vi "ADAM_Comparitor.vi"(3 "Comparator Info":T1, 4 "Ch names":string[](array[string]), 5 "Present scan array":dbl[](array[numeric]) format="%.2f") -> (0 "Comparator Info Out":T1, 2 "Scan comment":string)   [LabVIEW 2010]
uses:
  ADAM_Comparitor.ctl
  ADAM Client/Sub VIs/ADAM Controls/Search_mode.ctl
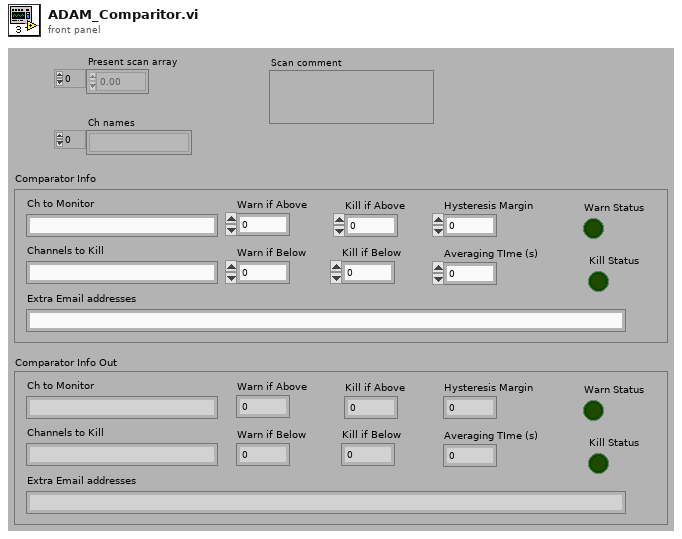
[diagram p1: front panel]
types:
  T1 = typedef "ADAM_Comparitor.ctl" = cluster{"Ch to Monitor":string, "Channels to Kill":string, "Warn if Above":dbl, "Warn if Below":dbl, "Kill if Above":dbl, "Kill if Below":dbl, "Hysteresis Margin":dbl, "Averaging TIme (s)":dbl, "Warn Status":bool, "Kill Status":bool, "Extra Email addresses":string}
  T2 = typedef "Search_mode.ctl" = enum16{"Between times", "All Times"}
  T3 = cluster{"Centre Times":dbl[], "Output array":dbl[]}
  T4 = cluster{"Centre Times":dbl[], "Output array":dbl[]}[]
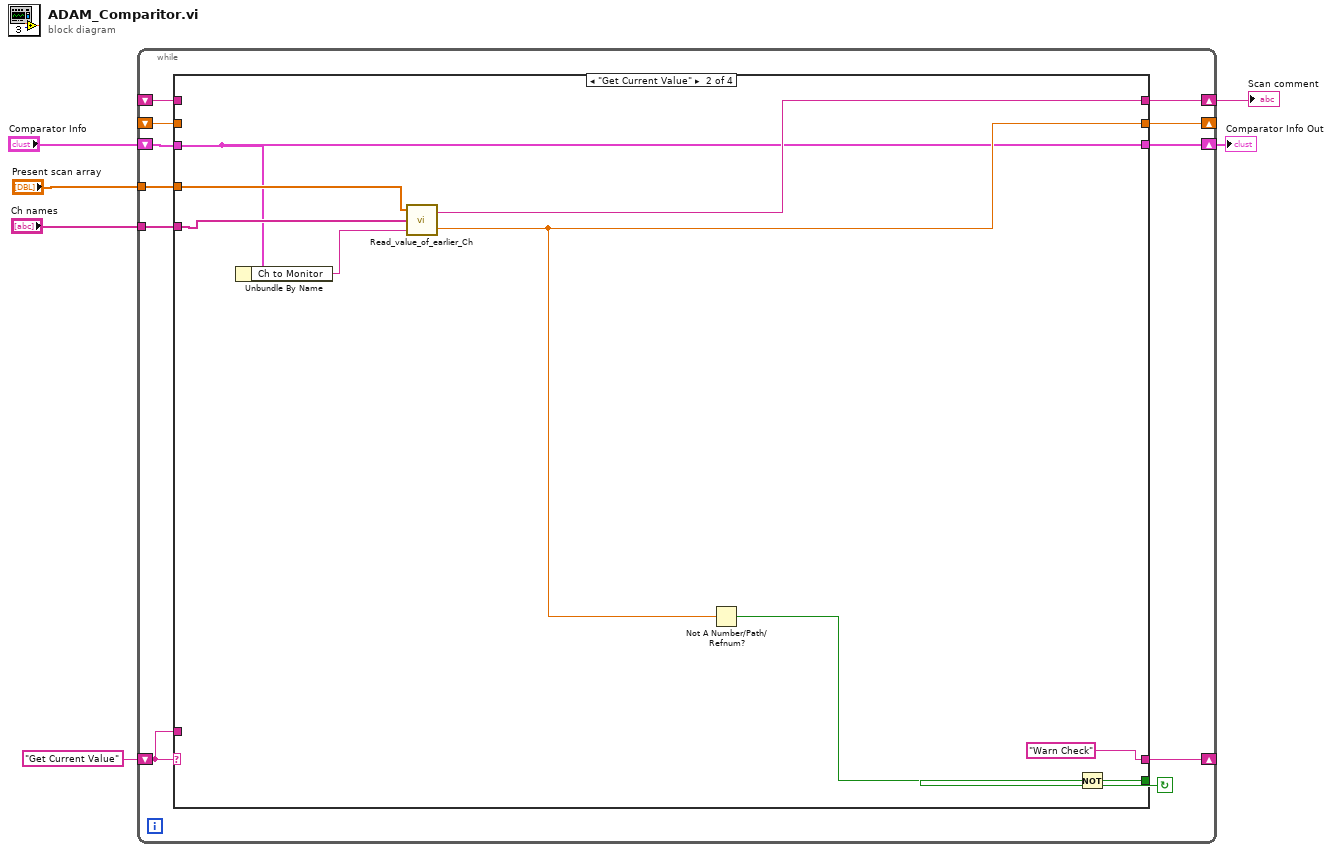
[diagram p0: block diagram]
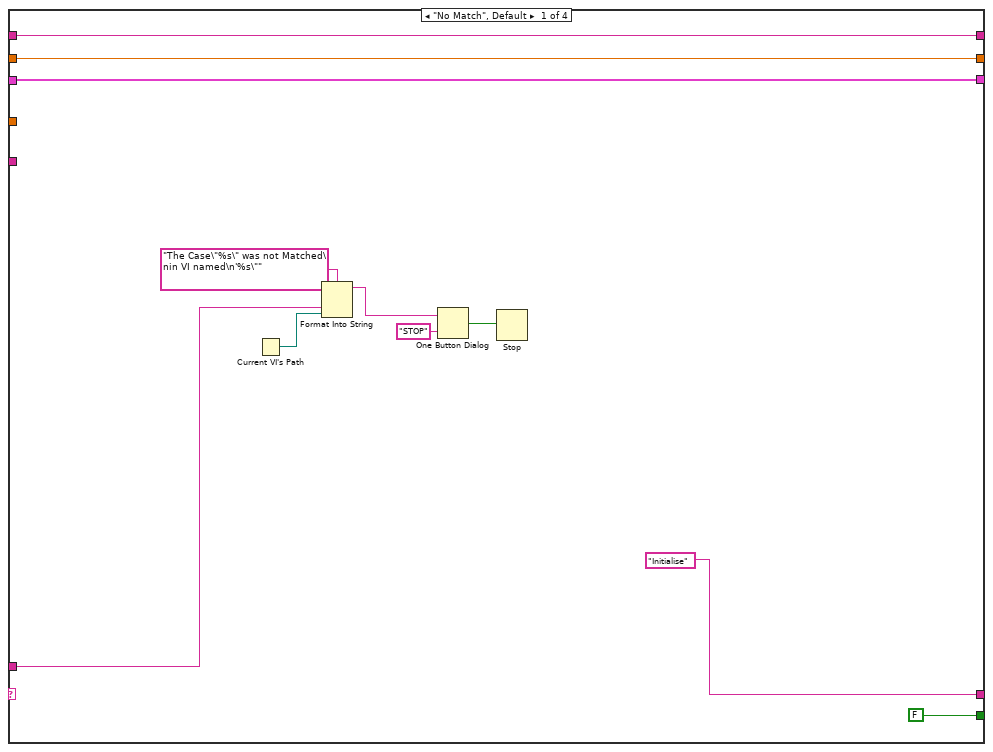
[diagram p2: hidden frame]
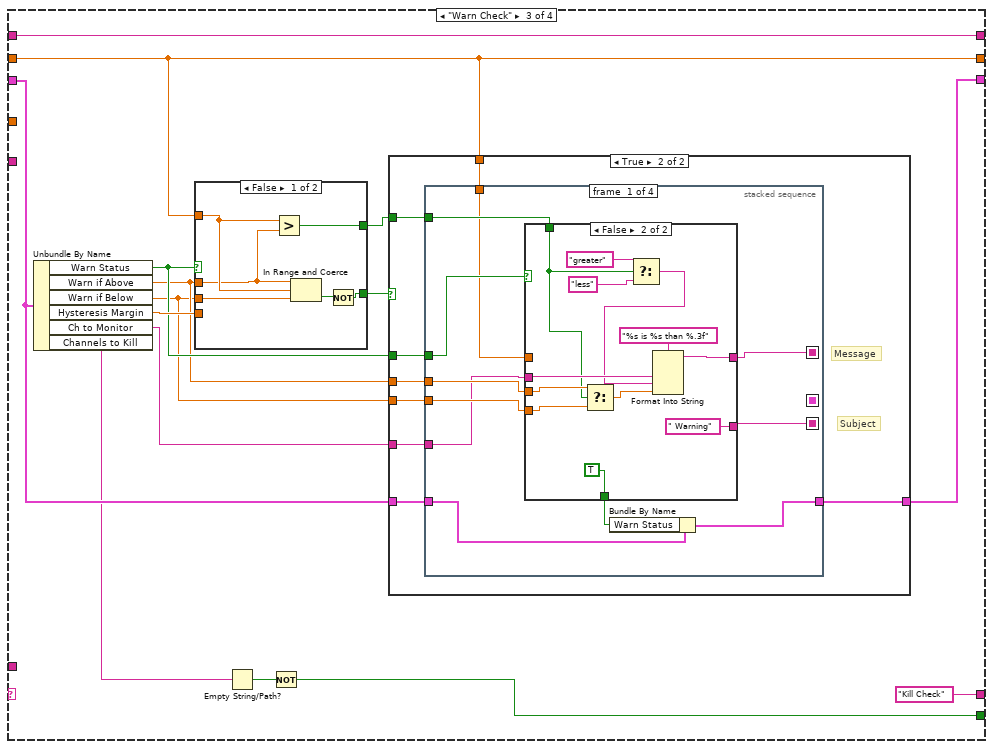
[diagram p3: hidden frame]
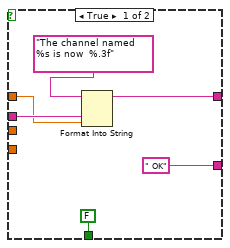
[diagram p5: hidden frame]
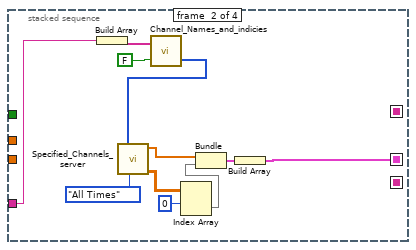
[diagram p6: hidden frame]
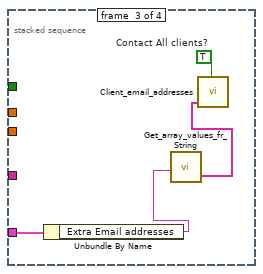
[diagram p7: hidden frame]
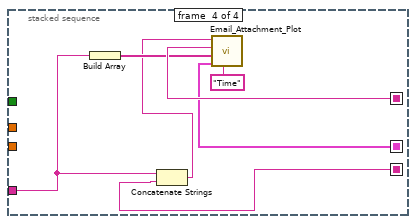
[diagram p8: hidden frame]
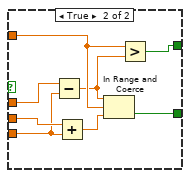
[diagram p9: hidden frame]
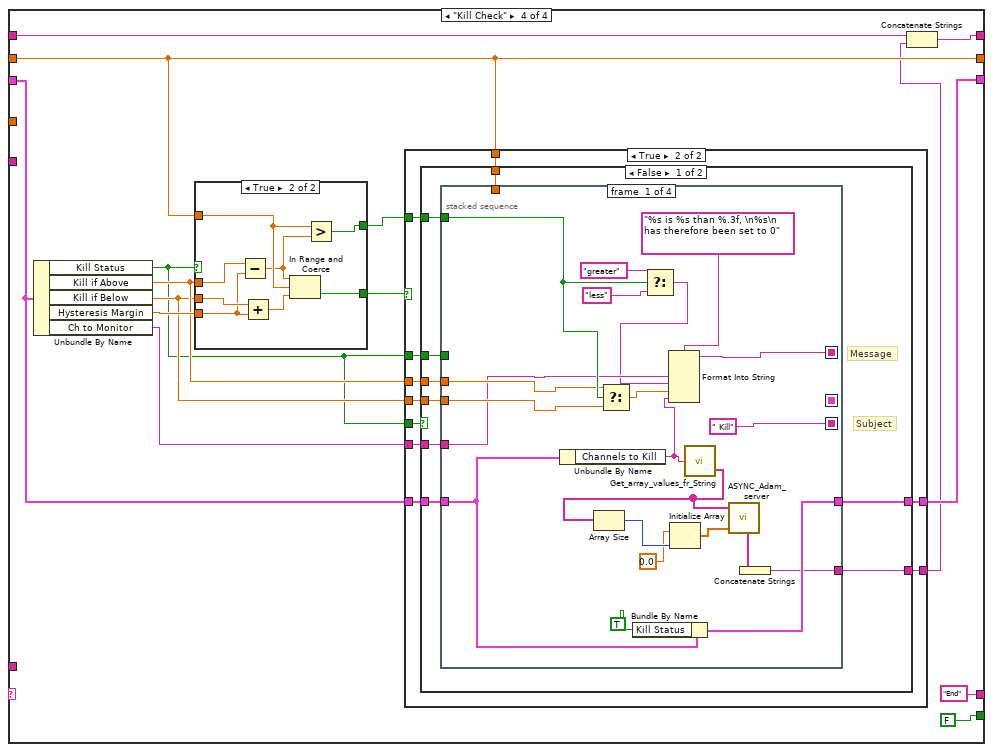
[diagram p10: hidden frame]
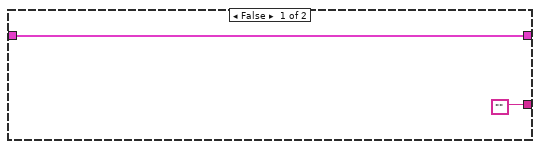
[diagram p11: hidden frame]
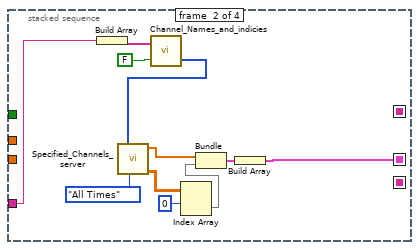
[diagram p12: hidden frame]
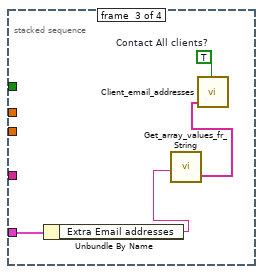
[diagram p13: hidden frame]
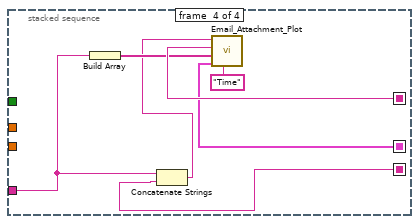
[diagram p14: hidden frame]
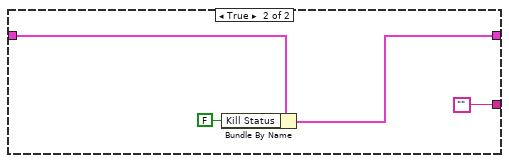
[diagram p15: hidden frame]
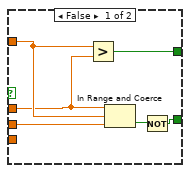
[diagram p16: hidden frame]
diagram:
  n1 = while {
    shift-left: "Get Current Value" -> [w15]
    shift-right: [w16] -> _
    tunnel: "Present scan array" -> [w14]
    tunnel: "Ch names" -> [w13]
    shift-right: [w10] -> w1
    shift-left: "Comparator Info" -> [w12]
    shift-right: [w11] -> _
    shift-left: _ -> [w9]
    shift-right: [w8] -> w2
    shift-left: _ -> [w7]
    stop <- w17 continue-if-true
    n2 = case shown="\"Get Current Value\"" w15 {
      tunnel: [FALSE w31 w40 FALSE] -> w17
      tunnel: ["Initialise" "Warn Check" "Kill Check" "End"] -> w16
      tunnel: w15 -> [w23 _ _ _]
      tunnel: w14 -> [_ w37 _ _]
      tunnel: w13 -> [_ w36 _ _]
      tunnel: w12 -> [w19 w29 w44 w134]
      tunnel: [w20 w33 w39 w132] -> w11
      tunnel: [w19 w29 w43 w133] -> w10
      tunnel: w9 -> [w20 _ w39 w132]
      tunnel: [w18 w34 w38 w129] -> w8
      tunnel: w7 -> [w18 _ w38 w130]
      frame "No Match", Default {
        n3 = Current VI's Path() -> (path=w22:path)
        n4 = Format Into String(format string="The Case\"%s\" was not Matched\nin VI named\n'%s\"" ("Format String"), w23, w22) -> (resulting string=w26:string)  [unwired: 2 in, 1 out]
        n5 = One Button Dialog(message=w26, button name ("OK")="STOP") -> (true=w24:bool)
        n6 = Stop(stop? (T)=w24) -> ()
      }
      frame "Get Current Value" {
        n7 = Unbundle By Name(w29) -> ("Ch to Monitor"=w35:string)
        n8 = call "Read_value_of_earlier_Ch.vi"("Desired Ch to Read"=w35, "Ch names"=w36, "Present scan array"=w37) -> ("Value"=w33:dbl, "Scan comment"=w34:string)  [unwired: 1 in]
        n9 = Not A Number/Path/Refnum?(number/path/refnum=w33) -> (NaN/Path/Refnum?=w32:bool)
        n10 = Not(x=w32) -> (.not. x?=w31:bool)
      }
      frame "Warn Check" {
        n11 = Unbundle By Name(w44) -> ("Warn Status"=w48:bool, "Warn if Above"=w47:dbl, "Warn if Below"=w46:dbl, "Hysteresis Margin"=w51:dbl, "Ch to Monitor"=w45:string, "Channels to Kill"=w42:string)
        n12 = case shown="False" w48 {
          tunnel: w47 -> [w117 w126]
          tunnel: w46 -> [w116 w125]
          tunnel: w39 -> [w118 w121]
          tunnel: w51 -> [_ w123]
          tunnel: [w114 w122] -> w50
          tunnel: [w113 w119] -> w49
          frame False {
            n13 = Greater?(x=w118, y=w117) -> (0:w113:bool)
            n14 = In Range and Coerce(upper limit=w117, x=w118, lower limit=w116) -> (In Range?=w115:bool)  [unwired: 1 out]
            n15 = Not(x=w115) -> (.not. x?=w114:bool)
          }
          frame True {
            n16 = Subtract(x=w126, y=w123) -> (x-y=w120:dbl)
            n17 = Add(x=w125, y=w123) -> (x+y=w124:dbl)
            n18 = In Range and Coerce(upper limit=w120, x=w121, lower limit=w124) -> (In Range?=w122:bool)  [unwired: 1 out]
            n19 = Greater?(x=w121, y=w120) -> (0:w119:bool)
          }
        }
        n20 = Empty String/Path?(string/path=w42) -> (empty?=w41:bool)
        n21 = Not(x=w41) -> (.not. x?=w40:bool)
        n22 = case shown="True" w50 {
          tunnel: w49 -> [_ w61]
          tunnel: w47 -> [_ w60]
          tunnel: w46 -> [_ w59]
          tunnel: w44 -> [w53 w58]
          tunnel: w48 -> [_ w57]
          tunnel: w39 -> [_ w56]
          tunnel: w45 -> [_ w55]
          tunnel: [w53 w54] -> w43
          frame False {
          }
          frame True {
            # "Subject"
            # "Message"
            n23 = stacked-sequence {
              seq-local: [w66 _ _ _] -> [_ _ _ w112]
              seq-local: [_ w93 _ _] -> [_ _ _ w110]
              seq-local: [w65 _ _ _] -> [_ _ _ w106]
              tunnel: w60 -> [w70 _ _ _]
              tunnel: w59 -> [w69 _ _ _]
              tunnel: w61 -> [w72 _ _ _]
              tunnel: w58 -> [w64 _ w103 _]
              tunnel: w57 -> [w71 _ _ _]
              tunnel: w56 -> [w68 _ _ _]
              tunnel: w55 -> [w67 w91 _ w107]
              tunnel: [w63 _ _ _] -> w54
              frame #0 {
                n24 = case shown="False" w71 {
                  tunnel: w67 -> [w78 w90]
                  tunnel: w70 -> [_ w84]
                  tunnel: [w76 w89] -> w66
                  tunnel: w69 -> [_ w83]
                  tunnel: [" OK" " Warning"] -> w65
                  tunnel: w68 -> [w74 _]
                  tunnel: w72 -> [_ w81]
                  tunnel: [FALSE ("Warn Status") TRUE ("Warn Status")] -> w62
                  frame True {
                    n25 = Format Into String(format string="The channel named %s is now  %.3f" ("Format String"), w78, w74) -> (resulting string=w76:string)  [unwired: 2 in, 1 out]
                  }
                  frame False {
                    n26 = Select(t=w84, s=w81, f=w83) -> (s? t:f=w82:dbl)
                    n27 = Select(t="greater", s=w81, f="less") -> (s? t:f=w85:string)
                    n28 = Format Into String(format string="%s is %s than %.3f" ("Format String"), w90, w85, w82) -> (resulting string=w89:string)  [unwired: 2 in, 1 out]
                  }
                }
                n29 = Bundle By Name(cluster=w64, "Warn Status"=w62) -> (w63:T1)
              }
              frame #1 {
                n30 = Build Array(w91) -> (w100:string[])
                n31 = call "Channel_Names_and_indicies.vi"("All Active Channels"=FALSE, "Desired Ch Names"=w100) -> ("Indicies"=w98:i32[])  [unwired: 1 out]
                n32 = call "Specified_Channels_server.vi"("Mode"=Search_mode."All Times", "Requested channels"=w98) -> ("Output array"=w96:dbl[][], "Centre Times"=w92:dbl[])  [unwired: 3 in, 3 out]
                n33 = Index Array(array=w96, index (row)=0) -> (element=w94:dbl[])  [unwired: 1 in]
                n34 = Bundle("Centre Times"=w92, "Output array"=w94) -> (w97:T3)  [unwired: 1 out]
                n35 = Build Array(w97) -> (w93:T4)
              }
              frame #2 {
                w105 = TRUE  # Contact All clients?
                n36 = Unbundle By Name(w103) -> ("Extra Email addresses"=w102:string)
                n37 = call "Get_array_values_fr_String.vi"("String Value"=w102) -> ("String array"=w104:string[])  [unwired: 1 out]
                n38 = call "Client_email_addresses.vi"("Extra People to Email"=w104, "Contact All clients?"=w105) -> ()  [unwired: 1 in]
              }
              frame #3 {
                n39 = Build Array(w107) -> (w111:string[])
                n40 = Concatenate Strings(w107, w106) -> (w108:string)
                n41 = call "Email_Attachment_Plot.vi"("X axis name"="Time", "XY Graph"=w110, "Series Names"=w111, "message"=w112, "subject ([No Subject])"=w108) -> ()  [unwired: 1 in, 1 out]
              }
            }
          }
        }
      }
      frame "Kill Check" {
        n42 = Unbundle By Name(w134) -> ("Kill Status"=w127:bool, "Kill if Above"=w137:dbl, "Kill if Below"=w136:dbl, "Hysteresis Margin"=w140:dbl, "Ch to Monitor"=w135:string)
        n43 = case shown="True" w127 {
          tunnel: w137 -> [w214 w223]
          tunnel: w136 -> [w213 w222]
          tunnel: w132 -> [w215 w218]
          tunnel: w140 -> [_ w220]
          tunnel: [w211 w219] -> w139
          tunnel: [w210 w216] -> w138
          frame False {
            n44 = Greater?(x=w215, y=w214) -> (0:w210:bool)
            n45 = In Range and Coerce(upper limit=w214, x=w215, lower limit=w213) -> (In Range?=w212:bool)  [unwired: 1 out]
            n46 = Not(x=w212) -> (.not. x?=w211:bool)
          }
          frame True {
            n47 = Subtract(x=w223, y=w220) -> (x-y=w217:dbl)
            n48 = Add(x=w222, y=w220) -> (x+y=w221:dbl)
            n49 = In Range and Coerce(upper limit=w217, x=w218, lower limit=w221) -> (In Range?=w219:bool)  [unwired: 1 out]
            n50 = Greater?(x=w218, y=w217) -> (0:w216:bool)
          }
        }
        n51 = case shown="True" w139 {
          tunnel: w138 -> [_ w153]
          tunnel: w137 -> [_ w152]
          tunnel: w136 -> [_ w151]
          tunnel: w134 -> [w143 w150]
          tunnel: w127 -> [_ w149]
          tunnel: w132 -> [_ w148]
          tunnel: w135 -> [_ w147]
          tunnel: [w143 w146] -> w133
          tunnel: ["" w145] -> w131
          tunnel: w127 -> [_ w144]
          frame False {
          }
          frame True {
            n52 = case shown="False" w144 {
              tunnel: w153 -> [w162 _]
              tunnel: w152 -> [w161 _]
              tunnel: w151 -> [w160 _]
              tunnel: w150 -> [w159 w209]
              tunnel: w149 -> [w158 _]
              tunnel: w148 -> [w157 _]
              tunnel: w147 -> [w156 _]
              tunnel: [w155 w208] -> w146
              tunnel: [w154 ""] -> w145
              frame False {
                # "Subject"
                # "Message"
                n53 = stacked-sequence {
                  seq-local: [w179 _ _ _] -> [_ _ _ w205]
                  seq-local: [_ w186 _ _] -> [_ _ _ w203]
                  seq-local: [" Kill" _ _ _] -> [_ _ _ w199]
                  tunnel: w161 -> [w182 _ _ _]
                  tunnel: w160 -> [w181 _ _ _]
                  tunnel: w162 -> [w183 _ _ _]
                  tunnel: w159 -> [w175 _ w196 _]
                  tunnel: w158 -> [_ _ _ _]
                  tunnel: w157 -> [_ _ _ _]
                  tunnel: w156 -> [w180 w184 _ w200]
                  tunnel: [w177 _ _ _] -> w155
                  tunnel: [w174 _ _ _] -> w154
                  frame #0 {
                    n54 = Unbundle By Name(w175) -> ("Channels to Kill"=w163:string)
                    n55 = Select(t=w182, s=w183, f=w181) -> (s? t:f=w169:dbl)
                    n56 = Bundle By Name(cluster=w175, "Kill Status"=TRUE ("Warn Status")) -> (w177:T1)
                    n57 = Select(t="greater", s=w183, f="less") -> (s? t:f=w170:string)
                    n58 = Format Into String(format string="%s is %s than %.3f, \n%s\n has therefore been set to 0" ("Format String"), w180, w170, w169, w163) -> (resulting string=w179:string)  [unwired: 2 in, 1 out]
                    n59 = call "Get_array_values_fr_String.vi"("String Value"=w163) -> ("String array"=w165:string[])  [unwired: 1 out]
                    n60 = Array Size(array=w165) -> (size(s)=w168:i32)
                    n61 = Initialize Array(0.0 ("y"), w168) -> (w167:dbl[])
                    n62 = call "ASYNC_Adam_server.vi"("Values"=w167, "Channel Names"=w165) -> ("Scan Comments"=w164:string[])  [unwired: 1 in, 2 out]
                    n63 = Concatenate Strings(w164) -> (w174:string)
                  }
                  frame #1 {
                    n64 = Build Array(w184) -> (w193:string[])
                    n65 = call "Channel_Names_and_indicies.vi"("All Active Channels"=FALSE, "Desired Ch Names"=w193) -> ("Indicies"=w191:i32[])  [unwired: 1 out]
                    n66 = call "Specified_Channels_server.vi"("Mode"=Search_mode."All Times", "Requested channels"=w191) -> ("Output array"=w189:dbl[][], "Centre Times"=w185:dbl[])  [unwired: 3 in, 3 out]
                    n67 = Index Array(array=w189, index (row)=0) -> (element=w187:dbl[])  [unwired: 1 in]
                    n68 = Bundle("Centre Times"=w185, "Output array"=w187) -> (w190:T3)  [unwired: 1 out]
                    n69 = Build Array(w190) -> (w186:T4)
                  }
                  frame #2 {
                    w198 = TRUE  # Contact All clients?
                    n70 = Unbundle By Name(w196) -> ("Extra Email addresses"=w195:string)
                    n71 = call "Get_array_values_fr_String.vi"("String Value"=w195) -> ("String array"=w197:string[])  [unwired: 1 out]
                    n72 = call "Client_email_addresses.vi"("Extra People to Email"=w197, "Contact All clients?"=w198) -> ()  [unwired: 1 in]
                  }
                  frame #3 {
                    n73 = Build Array(w200) -> (w204:string[])
                    n74 = Concatenate Strings(w200, w199) -> (w201:string)
                    n75 = call "Email_Attachment_Plot.vi"("X axis name"="Time", "XY Graph"=w203, "Series Names"=w204, "message"=w205, "subject ([No Subject])"=w201) -> ()  [unwired: 1 in, 1 out]
                  }
                }
              }
              frame True {
                n76 = Bundle By Name(cluster=w209, "Kill Status"=FALSE) -> (w208:T1)
              }
            }
          }
        }
        n77 = Concatenate Strings(w130, w131) -> (w129:string)
      }
    }
  }
  "Scan comment" <- w2
  "Comparator Info Out" <- w1
